vi "myRIO_BRig_Host_TCP_parseCmd_selectResponse__v2.vi"(10 "input_countCmd":i32, 11 "input_strCmd":string) -> (0 "output_countTrial":i32, 1 "output_L/R":i32, 2 "output_iTrial":i32, 3 "output_iBlock":i32, 4 "output_response":i32)   [LabVIEW 2014]
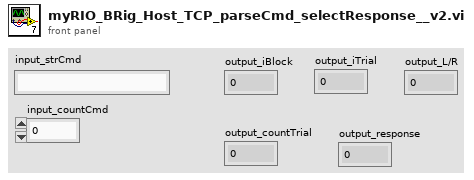
[diagram p1: front panel]
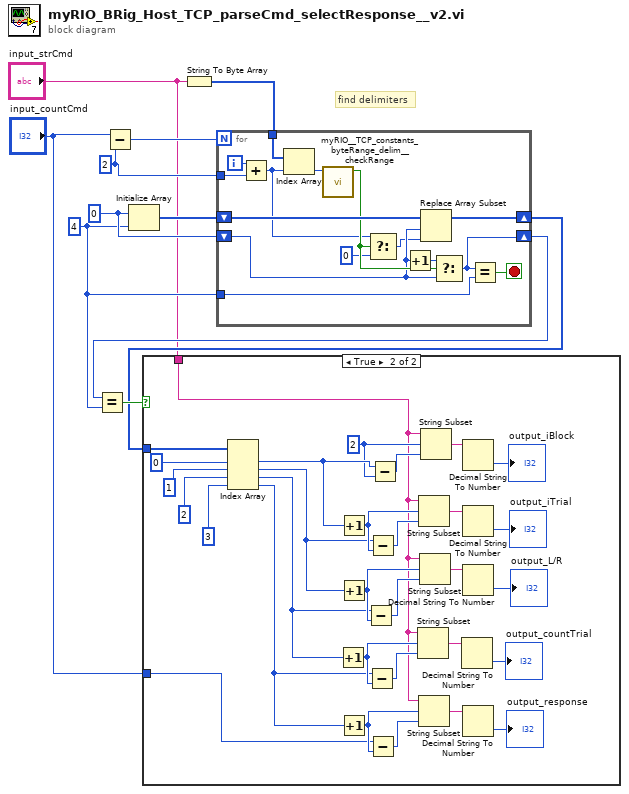
[diagram p0: block diagram]
diagram:
  w9 = 0 ("element")
  w3 = 4 ("dimension size")
  w10 = 2 ("y")
  # "find delimiters"
  n1 = Subtract(x="input_countCmd", y=w10) -> (x-y=w11:i32)
  n2 = Initialize Array(w9, w3) -> (w8:i32[])
  n3 = String To Byte Array(string="input_strCmd") -> (unsigned byte array=w7:u8[])
  n4 = for {
    N: w11 -> [_]
    tunnel: w10 -> [w25]
    shift-right: [w15] -> w6
    shift-left: w9 -> [w17]
    shift-right: [w12] -> w4
    shift-left: w8 -> [w24]
    tunnel: w7 -> [w23]
    tunnel: w3 -> [w14]
    i -> [w26]
    stop <- w13 stop-if-true
    n5 = Add(x=w26, y=w25) -> (x+y=w20:i32)
    n6 = Index Array(array=w23, index=w20) -> (element=w22:u8)
    n7 = call "myRIO__TCP_constants_byteRange_delim__checkRange.vi"("input_byte"=w22) -> ("output_delim"=w21:bool)  [unwired: 9 in, 1 out]
    n8 = Select(t=w20, s=w21, f=0) -> (s? t:f=w16:i32)
    n9 = Increment(x=w17) -> (x+1=w18:i32)
    n10 = Replace Array Subset(array=w24, new element=w16, index=w17) -> (w12:i32[])
    n11 = Select(t=w18, s=w21, f=w17) -> (s? t:f=w15:i32)
    n12 = Equal?(x=w15, y=w14) -> (x = y?=w13:bool)
  }
  n13 = Equal?(x=w6, y=w3) -> (x = y?=w5:bool)
  n14 = case shown="True" w5 {
    tunnel: w4 -> [_ w57]
    tunnel: "input_strCmd" -> [_ w27]
    tunnel: "input_countCmd" -> [_ w28]
    frame False {
    }
    frame True {
      w43 = 2 ("offset (0)")
      n15 = Index Array(array=w57, index #1=0 ("index"), index #2=1 ("index"), index #3=2 ("index"), index #4=3 ("index")) -> (element #1=w44:i32, element #2=w37:i32, element #3=w36:i32, element #4=w29:i32)
      n16 = Increment(x=w36) -> (x+1=w50:i32)
      n17 = Increment(x=w44) -> (x+1=w45:i32)
      n18 = Increment(x=w37) -> (x+1=w56:i32)
      n19 = Increment(x=w29) -> (x+1=w31:i32)
      n20 = Subtract(x=w36, y=w56) -> (x-y=w55:i32)
      n21 = Subtract(x=w29, y=w50) -> (x-y=w52:i32)
      n22 = Subtract(x=w37, y=w45) -> (x-y=w47:i32)
      n23 = Subtract(x=w28, y=w31) -> (x-y=w33:i32)
      n24 = Subtract(x=w44, y=w43) -> (x-y=w42:i32)
      n25 = String Subset(string=w27, offset (0)=w50, length (rest)=w52) -> (substring=w51:string)
      n26 = String Subset(string=w27, offset (0)=w45, length (rest)=w47) -> (substring=w46:string)
      n27 = String Subset(string=w27, offset (0)=w31, length (rest)=w33) -> (substring=w32:string)
      n28 = String Subset(string=w27, offset (0)=w56, length (rest)=w55) -> (substring=w54:string)
      n29 = String Subset(string=w27, offset (0)=w43, length (rest)=w42) -> (substring=w41:string)
      n30 = Decimal String To Number(string=w51) -> (number=→"output_countTrial":i32)  [unwired: 2 in, 1 out]
      n31 = Decimal String To Number(string=w41) -> (number=→"output_iBlock":i32)  [unwired: 2 in, 1 out]
      n32 = Decimal String To Number(string=w46) -> (number=→"output_iTrial":i32)  [unwired: 2 in, 1 out]
      n33 = Decimal String To Number(string=w54) -> (number=→"output_L/R":i32)  [unwired: 2 in, 1 out]
      n34 = Decimal String To Number(string=w32) -> (number=→"output_response":i32)  [unwired: 2 in, 1 out]
    }
  }
